vi "DHE_Callback.vi"(2 "DHE_InitMacro":path) -> ()   [LabVIEW 2016]
uses:
  DHE_GBLDriverVariables.vi
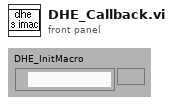
[diagram p1: front panel]
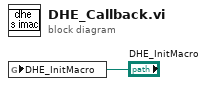
[diagram p0: block diagram]
diagram:
  n1 = global write "DHE_GBLDriverVariables.vi" "DHE_InitMacro"("DHE_InitMacro") -> ()
